vi "Choreo_TrajectoryDifferential_GetTotalTime.vi"(11 "ChoreoTrajectoryDifferential":T1) -> (3 "TotalTime":dbl)   [LabVIEW 2019, in "ChoreoLib.lvlib"]
doc: "Returns the total time of the trajectory (the timestamp of the last sample). This will return 0 if the trajectory is empty.\n\nInputs: \n - ChoreoTrajectory - cluster - Input trajectory\n\nOutputs:\n - TotalTime - double - The total time duration of this trajectory (seconds).\n."
uses:
  ChoreoLib.lvlib
  TypeDef/ChoreoTrajectoryDifferential.ctl
  TypeDef/ChoreoDifferentialSample.ctl
  TypeDef/ChoreoEventMarker.ctl
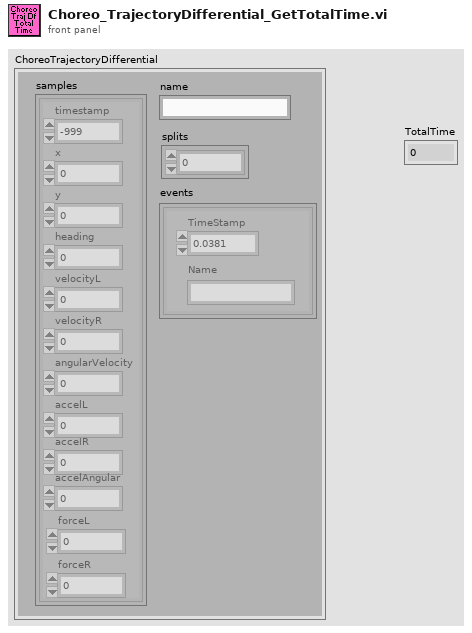
[diagram p1: front panel]
types:
  T1 = typedef "ChoreoLib.lvlib/ChoreoTrajectoryDifferential.ctl" = cluster{"name":string, "samples":T2[], "splits":i32[], "events":T3[]}
  T2 = typedef "ChoreoLib.lvlib/ChoreoDifferentialSample.ctl" = cluster{"timestamp":dbl, "x":dbl, "y":dbl, "heading":dbl, "velocityL":dbl, "velocityR":dbl, "angularVelocity":dbl, "accelL":dbl, "accelR":dbl, "accelAngular":dbl, "forceL":dbl, "forceR":dbl}
  T3 = typedef "ChoreoLib.lvlib/ChoreoEventMarker.ctl" = cluster{"TimeStamp":dbl, "Name":string}
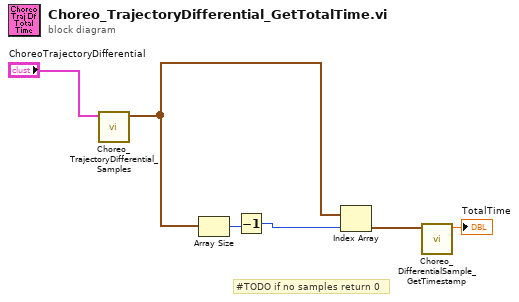
[diagram p0: block diagram]
diagram:
  # "#TODO if no samples return 0"
  n1 = call "Choreo_TrajectoryDifferential_Samples.vi"("ChoreoTrajectoryDifferential"="ChoreoTrajectoryDifferential") -> ("samples"=w1:T2[])  [unwired: 10 in]
  n2 = Array Size(array=w1) -> (size(s)=w6:i32)
  n3 = Decrement(x=w6) -> (x-1=w5:i32)
  n4 = Index Array(array=w1, index=w5) -> (element=w4:T2)
  n5 = call "Choreo_DifferentialSample_GetTimestamp.vi"("ChoreoDifferentialSample"=w4) -> ("Timestamp"=→"TotalTime":dbl)  [unwired: 10 in]
